vi "ADIS16470 IMU Calibration.vi"() -> ()   [LabVIEW 2017]
uses:
  <vilib>/Rock Robotics/SystemInterfaces/spilib/spi_bus.ctl
  <vilib>/Rock Robotics/SystemInterfaces/DIO/FPGA_DIOChannel.ctl
  <vilib>/Rock Robotics/WPI/SPI/WPI_SPIMode.ctl
  ADIS16448 IMU/ADI_IMU_ADIS16470_Registers.ctl
  ADIS16448 IMU/ADIS16470_IMU.lvlib
panel:
  in  "Operation":enum16{"Clear", "Read", "Calibrate"}(ring)=enum."Calibrate"
  out "Timer":dbl
  in  "SPI Chip Select":T1=enum."SPI MXP"
  out "Offset Registers":T2 {"zGYRO_OFF" format="%x"; "yGYRO_OFF" format="%x"; "xGYRO_OFF" format="%x"}
  out "Write Successful?":bool
  out "Device Found":bool
  # "FRC Analog Devices ADIS16448 IMU\nOffset Calibration Program"
  # "Instructions: \n* Place your robot in a stable location where it will not be bumped or moved.\n* Make sure that the IMU is securely mounted to the RoboRIO! \n* When ready, start the VI. The program will enable averaging inside of the IMU and will calculate the bias offset. \n* After recording data, the VI will save the data within the sensor for future use. \n* Running this utility again will overwrite the bias correction. \n* Running offset calibration (not this program) before a match is still recommended even after running this utility!"
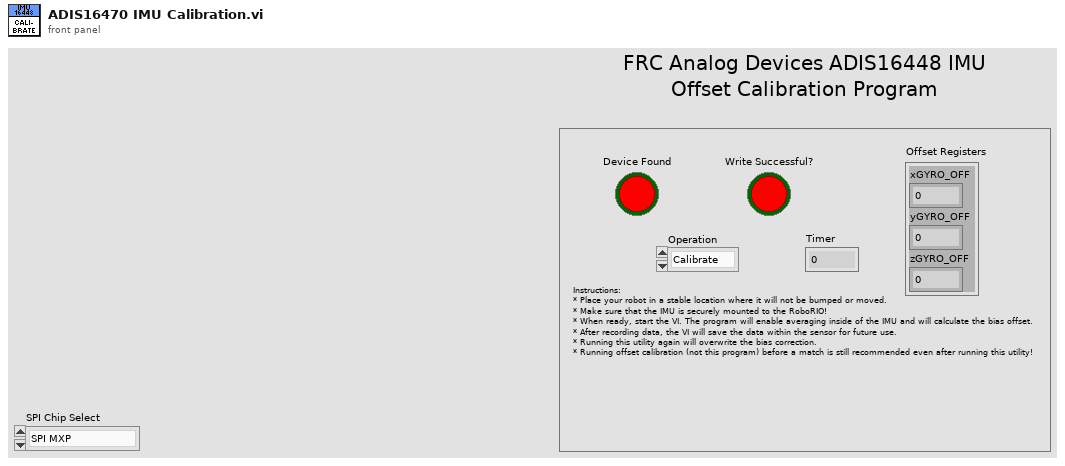
[diagram p1: front panel]
types:
  T1 = typedef "spi_bus.ctl" = enum16{"SPI On-Board, CS0", "SPI On-Board, CS1", "SPI On-Board, CS2", "SPI On-Board, CS3", "SPI MXP", "Invalid"}
  T2 = cluster{"xGYRO_OFF":u16, "yGYRO_OFF":u16, "zGYRO_OFF":u16}
  T3 = typedef "ADIS16470_IMU.lvlib/ADI_IMU_ADIS16470_Registers.ctl" = u8
  T4 = typedef "WPI_SPIMode.ctl" = enum16{"Mode 0 (Clk Idle Low,Sample on Leading)", "Mode 1 (Clk Idle Low,Sample on Trailing)", "Mode 2 (Clk Idle High,Sample on Leading)", "Mode 3 (Clk Idle High,Sample on Trailing)"}
  T5 = typedef "FPGA_DIOChannel.ctl" = enum8{"DIO 0", "DIO 1", "DIO 2", "DIO 3", "DIO 4", "DIO 5", "DIO 6", "DIO 7", "DIO 8", "DIO 9", "DIO MXP 0", "DIO MXP 1", "DIO MXP 2", "DIO MXP 3", "DIO MXP 4", "DIO MXP 5", "DIO MXP 6", "DIO MXP 7", "DIO MXP 8", "DIO MXP 9", "DIO MXP 10", "DIO MXP 11", "DIO MXP 12", "DIO MXP 13", "DIO MXP 14", "DIO MXP 15", "SPI Port CS1", "SPI Port CS2", "SPI Port CS3", "SPI Port MISO", "SPI Port MOSI", "Invalid"}
  T6 = typedef "WPI_DigitalOutputDevRef.ctl" = cluster{"DIO Channel":T5, "DevStatus":errorcluster}
  T7 = typedef "WPI_DigitalInputDevRef.ctl" = cluster{"DevStatus":errorcluster, "DIO Channel":T5}
  T8 = typedef "WPI_SPIDevRef.ctl" = cluster{"DevStatus":errorcluster, "Handle":i32, "SPI Bus":T1}
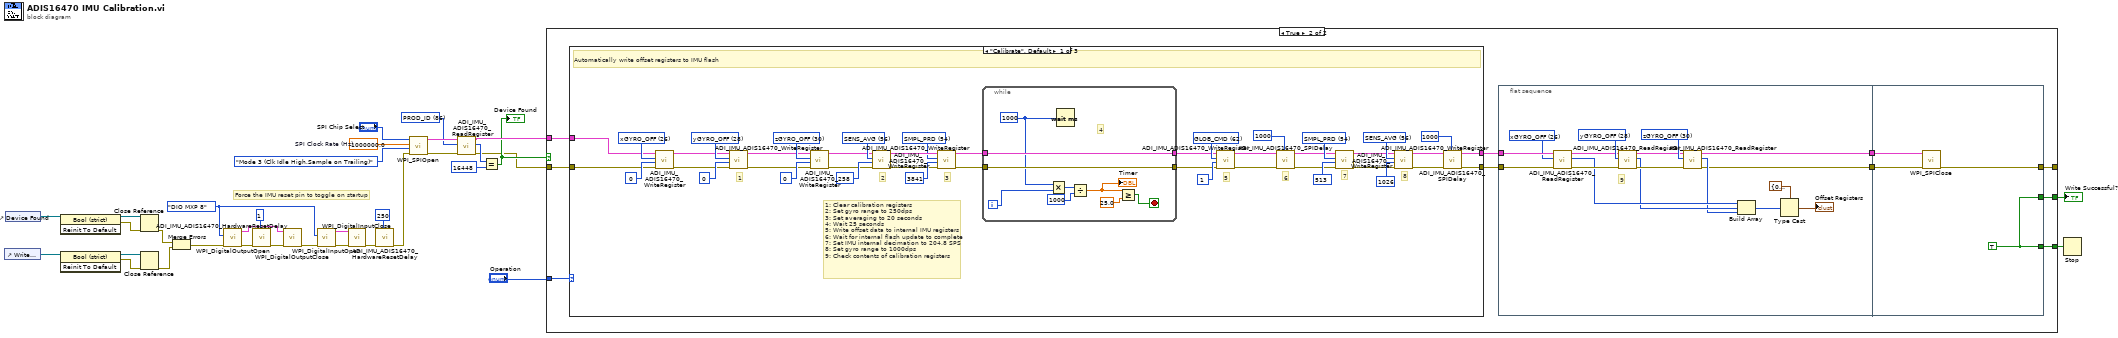
[diagram p0: block diagram]
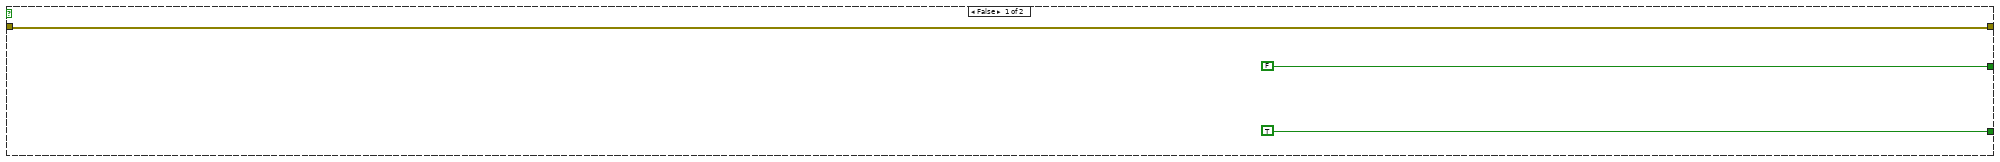
[diagram p2: hidden frame]
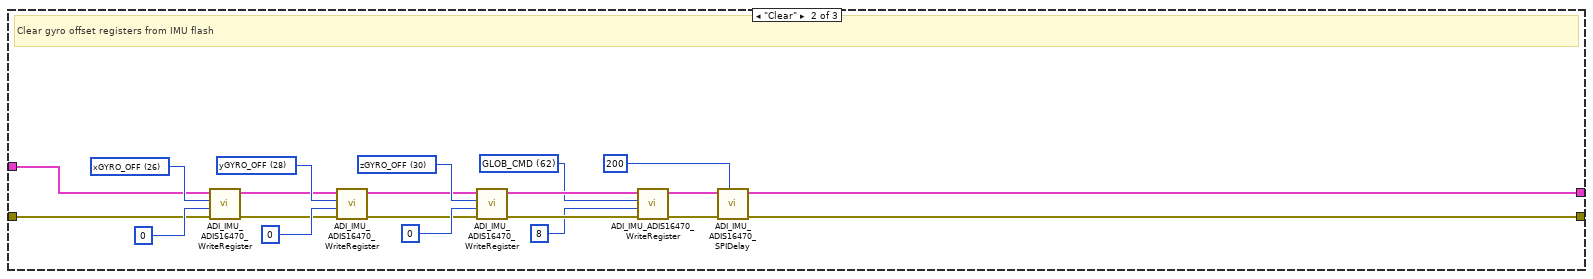
[diagram p3: hidden frame]
diagram:
  w15 = T3 86 items=["GLOB_CMD"=62, "SEQ_CNT"=58, "SMPL_PRD"=54, "SENS_AVG"=56, "MSC_CTRL"=52, "ERROR_FLAGS"=60, "TEMP"=44, "BARO"=40, "Z_MAG"=36, "Y_MAG"=32, "X_MAG"=28, "Z_ACCEL"=24, "Y_ACCEL"=20, "X_ACCEL"=16, "Z_GYRO"=12, "Y_GYRO"=8, "X_GYRO"=4, "PROD_ID"=86, "LOT_ID2"=84, "LOT_ID1"=82, "SERIAL_NUM"=88] ("ADIS16448 Register")
  w17 = 1000000.0  # SPI Clock Rate (Hz)
  w23 = FPGA_DIOChannel."DIO MXP 8" ("DIO Channel")
  # "Force the IMU reset pin to toggle on startup"
  n1 = control-ref of="Write Successful?"() -> (w4:refnum<vi>)
  n2 = control-ref of="Device Found"() -> (w7:refnum<vi>)
  n3 = invoke class="Bool (strict)" method="Reinit To Default"(reference=w7) -> (reference out=w9:refnum<vi>, error out=w8:errorcluster)  [unwired: 2 in, 1 out]
  n4 = invoke class="Bool (strict)" method="Reinit To Default"(reference=w4) -> (reference out=w6:refnum<vi>, error out=w5:errorcluster)  [unwired: 2 in, 1 out]
  n5 = Close Reference(reference=w9, error in (no error)=w8) -> (error out=w3:errorcluster)
  n6 = Close Reference(reference=w6, error in (no error)=w5) -> (error out=w2:errorcluster)
  n7 = Merge Errors(w3, w2) -> (w1:errorcluster)
  n8 = call <vilib>:"WPI_DigitalOutputOpen.vi"("error in (no error)"=w1, "DIO Channel"=w23) -> ("error out"=w30:errorcluster, "DigitalOutputDevRef"=w24:T6)  [unwired: 8 in]
  n9 = call "ADI_IMU_ADIS16470_HardwareResetDelay.vi"("Delay (ms)"=u32 1, "error in"=w30) -> ("error out"=w31:errorcluster)  [unwired: 9 in]
  n10 = call <vilib>:"WPI_DigitalOutputClose.vi"("error in (no error)"=w31, "DigitalOutputDevRef"=w24) -> ("error out"=w29:errorcluster)  [unwired: 9 in]
  n11 = call <vilib>:"WPI_DigitalInputOpen.vi"("error in (no error)"=w29, "DIO Channel"=w23) -> ("error out"=w28:errorcluster, "DigitalInputDevRef"=w27:T7)  [unwired: 8 in]
  n12 = call <vilib>:"WPI_DigitalInputClose.vi"("error in (no error)"=w28, "DigitalInputDevRef"=w27) -> ("error out"=w26:errorcluster)  [unwired: 9 in]
  n13 = call "ADI_IMU_ADIS16470_HardwareResetDelay.vi"("Delay (ms)"=u32 250, "error in"=w26) -> ("error out"=w12:errorcluster)  [unwired: 9 in]
  n14 = call <vilib>:"WPI_SPIOpen.vi"("error in"=w12, "Mode (3)"=WPI_SPIMode."Mode 3 (Clk Idle High,Sample on Trailing)", "Clock Rate (Hz)"=w17, "SPI Bus"="SPI Chip Select") -> ("error out"=w21:errorcluster, "SPIDevRef"=w22:T8)  [unwired: 6 in]
  n15 = call "ADI_IMU_ADIS16470_ReadRegister.vi"("error in (no error)"=w21, "ADIS16448 Register"=w15, "SPIDevRef in"=w22) -> ("error out"=w11:errorcluster, "Register Value"=w20:u16, "SPIDevRef out"=w14:T8)  [unwired: 6 in]
  n16 = Equal?(x=w20, y=u16 16448) -> (x = y?=w13:bool)
  "Device Found" <- w13
  n17 = case shown="True" w13 {
    tunnel: w14 -> [_ w47]
    tunnel: w11 -> [w35 w46]
    tunnel: [TRUE w45] -> w34
    tunnel: [FALSE w44] -> w33
    tunnel: "Operation" -> [_ w41]
    tunnel: [w35 w38] -> _
    frame False {
    }
    frame True {
      n18 = case shown="\"Calibrate\", Default" w41 {
        tunnel: w47 -> [w54 w109 w121]
        tunnel: w46 -> [w53 w108 w120]
        tunnel: [w48 w100 w121] -> w43
        tunnel: [w49 w99 w120] -> w42
        frame "Calibrate", Default {
          w61 = T3 30 items=["zGYRO_OFF"=30, "yGYRO_OFF"=28, "xGYRO_OFF"=26, "GLOB_CMD"=62, "SEQ_CNT"=58, "SMPL_PRD"=54, "SENS_AVG"=56, "MSC_CTRL"=52, "zACCEL_OFF"=36, "yACCEL_OFF"=34, "xACCEL_OFF"=32, "ERROR_FLAGS"=60, "TEMP"=24, "BARO"=22, "Z_MAG"=20, "Y_MAG"=18, "X_MAG"=16, "Z_ACCEL"=14, "Y_ACCEL"=12, "X_ACCEL"=10, "Z_GYRO"=8, "Y_GYRO"=6, "X_GYRO"=4, "PROD_ID"=86, "LOT_ID2"=84, "LOT_ID1"=82, "SERIAL_NUM"=88] ("ADIS16448 Register")
          w64 = T3 28 items=["zGYRO_OFF"=30, "yGYRO_OFF"=28, "xGYRO_OFF"=26, "GLOB_CMD"=62, "SEQ_CNT"=58, "SMPL_PRD"=54, "SENS_AVG"=56, "MSC_CTRL"=52, "zACCEL_OFF"=36, "yACCEL_OFF"=34, "xACCEL_OFF"=32, "ERROR_FLAGS"=60, "TEMP"=24, "BARO"=22, "Z_MAG"=20, "Y_MAG"=18, "X_MAG"=16, "Z_ACCEL"=14, "Y_ACCEL"=12, "X_ACCEL"=10, "Z_GYRO"=8, "Y_GYRO"=6, "X_GYRO"=4, "PROD_ID"=86, "LOT_ID2"=84, "LOT_ID1"=82, "SERIAL_NUM"=88] ("ADIS16448 Register")
          w65 = T3 26 items=["zGYRO_OFF"=30, "yGYRO_OFF"=28, "xGYRO_OFF"=26, "GLOB_CMD"=62, "SEQ_CNT"=58, "SMPL_PRD"=54, "SENS_AVG"=56, "MSC_CTRL"=52, "zACCEL_OFF"=36, "yACCEL_OFF"=34, "xACCEL_OFF"=32, "ERROR_FLAGS"=60, "TEMP"=24, "BARO"=22, "Z_MAG"=20, "Y_MAG"=18, "X_MAG"=16, "Z_ACCEL"=14, "Y_ACCEL"=12, "X_ACCEL"=10, "Z_GYRO"=8, "Y_GYRO"=6, "X_GYRO"=4, "PROD_ID"=86, "LOT_ID2"=84, "LOT_ID1"=82, "SERIAL_NUM"=88] ("ADIS16448 Register")
          w78 = T3 54 items=["zGYRO_OFF"=30, "yGYRO_OFF"=28, "xGYRO_OFF"=26, "GLOB_CMD"=62, "SEQ_CNT"=58, "SMPL_PRD"=54, "SENS_AVG"=56, "MSC_CTRL"=52, "zACCEL_OFF"=36, "yACCEL_OFF"=34, "xACCEL_OFF"=32, "ERROR_FLAGS"=60, "TEMP"=24, "BARO"=22, "Z_MAG"=20, "Y_MAG"=18, "X_MAG"=16, "Z_ACCEL"=14, "Y_ACCEL"=12, "X_ACCEL"=10, "Z_GYRO"=8, "Y_GYRO"=6, "X_GYRO"=4, "PROD_ID"=86, "LOT_ID2"=84, "LOT_ID1"=82, "SERIAL_NUM"=88] ("ADIS16448 Register")
          w79 = T3 54 items=["zGYRO_OFF"=30, "yGYRO_OFF"=28, "xGYRO_OFF"=26, "GLOB_CMD"=62, "SEQ_CNT"=58, "SMPL_PRD"=54, "SENS_AVG"=56, "MSC_CTRL"=52, "zACCEL_OFF"=36, "yACCEL_OFF"=34, "xACCEL_OFF"=32, "ERROR_FLAGS"=60, "TEMP"=24, "BARO"=22, "Z_MAG"=20, "Y_MAG"=18, "X_MAG"=16, "Z_ACCEL"=14, "Y_ACCEL"=12, "X_ACCEL"=10, "Z_GYRO"=8, "Y_GYRO"=6, "X_GYRO"=4, "PROD_ID"=86, "LOT_ID2"=84, "LOT_ID1"=82, "SERIAL_NUM"=88] ("ADIS16448 Register")
          w81 = T3 62 items=["zGYRO_OFF"=30, "yGYRO_OFF"=28, "xGYRO_OFF"=26, "GLOB_CMD"=62, "SEQ_CNT"=58, "SMPL_PRD"=54, "SENS_AVG"=56, "MSC_CTRL"=52, "zACCEL_OFF"=36, "yACCEL_OFF"=34, "xACCEL_OFF"=32, "ERROR_FLAGS"=60, "TEMP"=24, "BARO"=22, "Z_MAG"=20, "Y_MAG"=18, "X_MAG"=16, "Z_ACCEL"=14, "Y_ACCEL"=12, "X_ACCEL"=10, "Z_GYRO"=8, "Y_GYRO"=6, "X_GYRO"=4, "PROD_ID"=86, "LOT_ID2"=84, "LOT_ID1"=82, "SERIAL_NUM"=88] ("ADIS16448 Register")
          w84 = T3 56 items=["GLOB_CMD"=62, "SEQ_CNT"=58, "SMPL_PRD"=54, "SENS_AVG"=56, "MSC_CTRL"=52, "ERROR_FLAGS"=60, "TEMP"=44, "BARO"=40, "Z_MAG"=36, "Y_MAG"=32, "X_MAG"=28, "Z_ACCEL"=24, "Y_ACCEL"=20, "X_ACCEL"=16, "Z_GYRO"=12, "Y_GYRO"=8, "X_GYRO"=4, "PROD_ID"=86, "LOT_ID2"=84, "LOT_ID1"=82, "SERIAL_NUM"=88] ("ADIS16448 Register")
          w89 = T3 56 items=["GLOB_CMD"=62, "SEQ_CNT"=58, "SMPL_PRD"=54, "SENS_AVG"=56, "MSC_CTRL"=52, "ERROR_FLAGS"=60, "TEMP"=44, "BARO"=40, "Z_MAG"=36, "Y_MAG"=32, "X_MAG"=28, "Z_ACCEL"=24, "Y_ACCEL"=20, "X_ACCEL"=16, "Z_GYRO"=12, "Y_GYRO"=8, "X_GYRO"=4, "PROD_ID"=86, "LOT_ID2"=84, "LOT_ID1"=82, "SERIAL_NUM"=88] ("ADIS16448 Register")
          # "8"
          # "1"
          # "7"
          # "6"
          # "5"
          # "3"
          # "2"
          # "1: Clear calibration registers\n2: Set gyro range to 250dps\n3: Set averaging to 20 seconds\n4: Wait 25 seconds\n5: Write offset data to internal IMU registers\n6: Wait for internal flash update to complete\n7: Set IMU internal decimation to 204.8 SPS \n8: Set gyro range to 1000dps\n9: Check contents of calibration registers"
          # "Automatically write offset registers to IMU flash"
          n19 = call "ADI_IMU_ADIS16470_WriteRegister.vi"("error in (no error)"=w53, "Data"=u16 0, "ADIS16448 Register"=w65, "SPIDevRef in"=w54) -> ("error out"=w57:errorcluster, "SPIDevRef out"=w58:T8)  [unwired: 6 in]
          n20 = call "ADI_IMU_ADIS16470_WriteRegister.vi"("error in (no error)"=w57, "Data"=u16 0, "ADIS16448 Register"=w64, "SPIDevRef in"=w58) -> ("error out"=w59:errorcluster, "SPIDevRef out"=w60:T8)  [unwired: 6 in]
          n21 = call "ADI_IMU_ADIS16470_WriteRegister.vi"("error in (no error)"=w59, "Data"=u16 0, "ADIS16448 Register"=w61, "SPIDevRef in"=w60) -> ("error out"=w55:errorcluster, "SPIDevRef out"=w56:T8)  [unwired: 6 in]
          n22 = call "ADI_IMU_ADIS16470_WriteRegister.vi"("error in (no error)"=w55, "Data"=u16 258, "ADIS16448 Register"=w89, "SPIDevRef in"=w56) -> ("error out"=w82:errorcluster, "SPIDevRef out"=w83:T8)  [unwired: 6 in]
          n23 = call "ADI_IMU_ADIS16470_WriteRegister.vi"("error in (no error)"=w82, "Data"=u16 3841, "ADIS16448 Register"=w78, "SPIDevRef in"=w83) -> ("error out"=w67:errorcluster, "SPIDevRef out"=w68:T8)  [unwired: 6 in]
          n24 = while {
            tunnel: [w96] -> w70
            tunnel: w67 -> [w96]
            tunnel: [w95] -> w69
            tunnel: w68 -> [w95]
            i -> [w93]
            stop <- w97 stop-if-true
            w94 = u32 1000 ("milliseconds to wait")
            # "4"
            n25 = Multiply(x=w94, y=w93) -> (x*y=w92:u32)
            n26 = Wait (ms)(milliseconds to wait=w94) -> ()  [unwired: 1 out]
            n27 = Divide(x=w92, y=u32 1000) -> (x/y=w90:dbl)
            "Timer" <- w90
            n28 = Greater Or Equal?(x=w90, y=25.0) -> (x >= y?=w97:bool)
          }
          n29 = call "ADI_IMU_ADIS16470_WriteRegister.vi"("error in (no error)"=w70, "Data"=u16 1, "ADIS16448 Register"=w81, "SPIDevRef in"=w69) -> ("error out"=w74:errorcluster, "SPIDevRef out"=w75:T8)  [unwired: 6 in]
          n30 = call "ADI_IMU_ADIS16470_SPIDelay.vi"("Wait (ms)"=u32 1000, "error in"=w74, "SPIDevRef in"=w75) -> ("error out"=w72:errorcluster, "SPIDevRef out"=w73:T8)  [unwired: 7 in]
          n31 = call "ADI_IMU_ADIS16470_WriteRegister.vi"("error in (no error)"=w72, "Data"=u16 513, "ADIS16448 Register"=w79, "SPIDevRef in"=w73) -> ("error out"=w76:errorcluster, "SPIDevRef out"=w77:T8)  [unwired: 6 in]
          n32 = call "ADI_IMU_ADIS16470_WriteRegister.vi"("error in (no error)"=w76, "Data"=u16 1026, "ADIS16448 Register"=w84, "SPIDevRef in"=w77) -> ("error out"=w50:errorcluster, "SPIDevRef out"=w51:T8)  [unwired: 6 in]
          n33 = call "ADI_IMU_ADIS16470_SPIDelay.vi"("Wait (ms)"=u32 1000, "error in"=w50, "SPIDevRef in"=w51) -> ("error out"=w49:errorcluster, "SPIDevRef out"=w48:T8)  [unwired: 7 in]
        }
        frame "Clear" {
          w105 = T3 62 items=["zGYRO_OFF"=30, "yGYRO_OFF"=28, "xGYRO_OFF"=26, "GLOB_CMD"=62, "SEQ_CNT"=58, "SMPL_PRD"=54, "SENS_AVG"=56, "MSC_CTRL"=52, "zACCEL_OFF"=36, "yACCEL_OFF"=34, "xACCEL_OFF"=32, "ERROR_FLAGS"=60, "TEMP"=24, "BARO"=22, "Z_MAG"=20, "Y_MAG"=18, "X_MAG"=16, "Z_ACCEL"=14, "Y_ACCEL"=12, "X_ACCEL"=10, "Z_GYRO"=8, "Y_GYRO"=6, "X_GYRO"=4, "PROD_ID"=86, "LOT_ID2"=84, "LOT_ID1"=82, "SERIAL_NUM"=88] ("ADIS16448 Register")
          w114 = T3 30 items=["zGYRO_OFF"=30, "yGYRO_OFF"=28, "xGYRO_OFF"=26, "GLOB_CMD"=62, "SEQ_CNT"=58, "SMPL_PRD"=54, "SENS_AVG"=56, "MSC_CTRL"=52, "zACCEL_OFF"=36, "yACCEL_OFF"=34, "xACCEL_OFF"=32, "ERROR_FLAGS"=60, "TEMP"=24, "BARO"=22, "Z_MAG"=20, "Y_MAG"=18, "X_MAG"=16, "Z_ACCEL"=14, "Y_ACCEL"=12, "X_ACCEL"=10, "Z_GYRO"=8, "Y_GYRO"=6, "X_GYRO"=4, "PROD_ID"=86, "LOT_ID2"=84, "LOT_ID1"=82, "SERIAL_NUM"=88] ("ADIS16448 Register")
          w117 = T3 28 items=["zGYRO_OFF"=30, "yGYRO_OFF"=28, "xGYRO_OFF"=26, "GLOB_CMD"=62, "SEQ_CNT"=58, "SMPL_PRD"=54, "SENS_AVG"=56, "MSC_CTRL"=52, "zACCEL_OFF"=36, "yACCEL_OFF"=34, "xACCEL_OFF"=32, "ERROR_FLAGS"=60, "TEMP"=24, "BARO"=22, "Z_MAG"=20, "Y_MAG"=18, "X_MAG"=16, "Z_ACCEL"=14, "Y_ACCEL"=12, "X_ACCEL"=10, "Z_GYRO"=8, "Y_GYRO"=6, "X_GYRO"=4, "PROD_ID"=86, "LOT_ID2"=84, "LOT_ID1"=82, "SERIAL_NUM"=88] ("ADIS16448 Register")
          w118 = T3 26 items=["zGYRO_OFF"=30, "yGYRO_OFF"=28, "xGYRO_OFF"=26, "GLOB_CMD"=62, "SEQ_CNT"=58, "SMPL_PRD"=54, "SENS_AVG"=56, "MSC_CTRL"=52, "zACCEL_OFF"=36, "yACCEL_OFF"=34, "xACCEL_OFF"=32, "ERROR_FLAGS"=60, "TEMP"=24, "BARO"=22, "Z_MAG"=20, "Y_MAG"=18, "X_MAG"=16, "Z_ACCEL"=14, "Y_ACCEL"=12, "X_ACCEL"=10, "Z_GYRO"=8, "Y_GYRO"=6, "X_GYRO"=4, "PROD_ID"=86, "LOT_ID2"=84, "LOT_ID1"=82, "SERIAL_NUM"=88] ("ADIS16448 Register")
          # "Clear gyro offset registers from IMU flash"
          n34 = call "ADI_IMU_ADIS16470_WriteRegister.vi"("error in (no error)"=w108, "Data"=u16 0, "ADIS16448 Register"=w118, "SPIDevRef in"=w109) -> ("error out"=w110:errorcluster, "SPIDevRef out"=w111:T8)  [unwired: 6 in]
          n35 = call "ADI_IMU_ADIS16470_WriteRegister.vi"("error in (no error)"=w110, "Data"=u16 0, "ADIS16448 Register"=w117, "SPIDevRef in"=w111) -> ("error out"=w112:errorcluster, "SPIDevRef out"=w113:T8)  [unwired: 6 in]
          n36 = call "ADI_IMU_ADIS16470_WriteRegister.vi"("error in (no error)"=w112, "Data"=u16 0, "ADIS16448 Register"=w114, "SPIDevRef in"=w113) -> ("error out"=w106:errorcluster, "SPIDevRef out"=w107:T8)  [unwired: 6 in]
          n37 = call "ADI_IMU_ADIS16470_WriteRegister.vi"("error in (no error)"=w106, "Data"=u16 8, "ADIS16448 Register"=w105, "SPIDevRef in"=w107) -> ("error out"=w101:errorcluster, "SPIDevRef out"=w102:T8)  [unwired: 6 in]
          n38 = call "ADI_IMU_ADIS16470_SPIDelay.vi"("Wait (ms)"=u32 200, "error in"=w101, "SPIDevRef in"=w102) -> ("error out"=w99:errorcluster, "SPIDevRef out"=w100:T8)  [unwired: 7 in]
        }
        frame "Read" {
        }
      }
      n39 = flat-sequence {
        tunnel: w43 -> [w138]
        tunnel: w42 -> [w137]
        tunnel: [w123] -> w40
        tunnel: [w122] -> w39
        tunnel: [w142] -> w45
        tunnel: [w142] -> w44
        tunnel: w40 -> [w141]
        tunnel: w39 -> [w140]
        tunnel: [w139] -> w38
        frame #0 {
          w134 = T3 30 items=["zGYRO_OFF"=30, "yGYRO_OFF"=28, "xGYRO_OFF"=26, "GLOB_CMD"=62, "SEQ_CNT"=58, "SMPL_PRD"=54, "SENS_AVG"=56, "MSC_CTRL"=52, "zACCEL_OFF"=36, "yACCEL_OFF"=34, "xACCEL_OFF"=32, "ERROR_FLAGS"=60, "TEMP"=24, "BARO"=22, "Z_MAG"=20, "Y_MAG"=18, "X_MAG"=16, "Z_ACCEL"=14, "Y_ACCEL"=12, "X_ACCEL"=10, "Z_GYRO"=8, "Y_GYRO"=6, "X_GYRO"=4, "PROD_ID"=86, "LOT_ID2"=84, "LOT_ID1"=82, "SERIAL_NUM"=88] ("ADIS16448 Register")
          w135 = T3 28 items=["zGYRO_OFF"=30, "yGYRO_OFF"=28, "xGYRO_OFF"=26, "GLOB_CMD"=62, "SEQ_CNT"=58, "SMPL_PRD"=54, "SENS_AVG"=56, "MSC_CTRL"=52, "zACCEL_OFF"=36, "yACCEL_OFF"=34, "xACCEL_OFF"=32, "ERROR_FLAGS"=60, "TEMP"=24, "BARO"=22, "Z_MAG"=20, "Y_MAG"=18, "X_MAG"=16, "Z_ACCEL"=14, "Y_ACCEL"=12, "X_ACCEL"=10, "Z_GYRO"=8, "Y_GYRO"=6, "X_GYRO"=4, "PROD_ID"=86, "LOT_ID2"=84, "LOT_ID1"=82, "SERIAL_NUM"=88] ("ADIS16448 Register")
          w136 = T3 26 items=["zGYRO_OFF"=30, "yGYRO_OFF"=28, "xGYRO_OFF"=26, "GLOB_CMD"=62, "SEQ_CNT"=58, "SMPL_PRD"=54, "SENS_AVG"=56, "MSC_CTRL"=52, "zACCEL_OFF"=36, "yACCEL_OFF"=34, "xACCEL_OFF"=32, "ERROR_FLAGS"=60, "TEMP"=24, "BARO"=22, "Z_MAG"=20, "Y_MAG"=18, "X_MAG"=16, "Z_ACCEL"=14, "Y_ACCEL"=12, "X_ACCEL"=10, "Z_GYRO"=8, "Y_GYRO"=6, "X_GYRO"=4, "PROD_ID"=86, "LOT_ID2"=84, "LOT_ID1"=82, "SERIAL_NUM"=88] ("ADIS16448 Register")
          # "9"
          n40 = call "ADI_IMU_ADIS16470_ReadRegister.vi"("error in (no error)"=w137, "ADIS16448 Register"=w136, "SPIDevRef in"=w138) -> ("error out"=w132:errorcluster, "Register Value"=w129:u16, "SPIDevRef out"=w133:T8)  [unwired: 6 in]
          n41 = call "ADI_IMU_ADIS16470_ReadRegister.vi"("error in (no error)"=w132, "ADIS16448 Register"=w135, "SPIDevRef in"=w133) -> ("error out"=w130:errorcluster, "Register Value"=w128:u16, "SPIDevRef out"=w131:T8)  [unwired: 6 in]
          n42 = call "ADI_IMU_ADIS16470_ReadRegister.vi"("error in (no error)"=w130, "ADIS16448 Register"=w134, "SPIDevRef in"=w131) -> ("error out"=w122:errorcluster, "Register Value"=w127:u16, "SPIDevRef out"=w123:T8)  [unwired: 6 in]
          n43 = Build Array(w129, w128, w127) -> (w126:u16[])
          n44 = Type Cast(type=T2 {"xGYRO_OFF"=0, "yGYRO_OFF"=0, "zGYRO_OFF"=0} ("Offset Registers 2"), x=w126) -> (*(type *) &x=→"Offset Registers":T2)
        }
        frame #1 {
          w142 = TRUE
          n45 = call <vilib>:"WPI_SPIClose.vi"("error in (no error)"=w140, "SPIDevRef"=w141) -> ("error out"=w139:errorcluster)  [unwired: 9 in]
        }
      }
    }
  }
  "Write Successful?" <- w33
  n46 = Stop(stop? (T)=w34) -> ()
